vi "Get Descriptor.vi"(0 "VISA resource name":refnum<visa-resource-name>, 5 "Source (1: Channel 1)":u16(ring)=1 items=["Channel 1"=1, "Channel 2"=2, "Channel 3"=3, "Channel 4"=4], 11 "error in (no error)":errorcluster) -> (1 "First Valid Point":i32, 2 "Last Valid Point":i32, 3 "Horizontal interval":sgl, 4 "VISA resource name out":refnum<visa-resource-name>, 6 "Vertical gain":sgl, 8 "Horizontal Offset":dbl, 10 "Vertical offset":sgl, 12 "Number Of Data Points":i32, 13 "Trigger Time":T1, 14 "Command type":i16, 15 "error out":errorcluster)   [LabVIEW 2021, in "Siglent SDS 1000 2000 Series.lvlib"]
doc: "Get basic information about acquisition waveform from specified channel."
uses:
  <instrlib>/Siglent SDS 1000 2000 Series/Siglent SDS 1000 2000 Series.lvlib
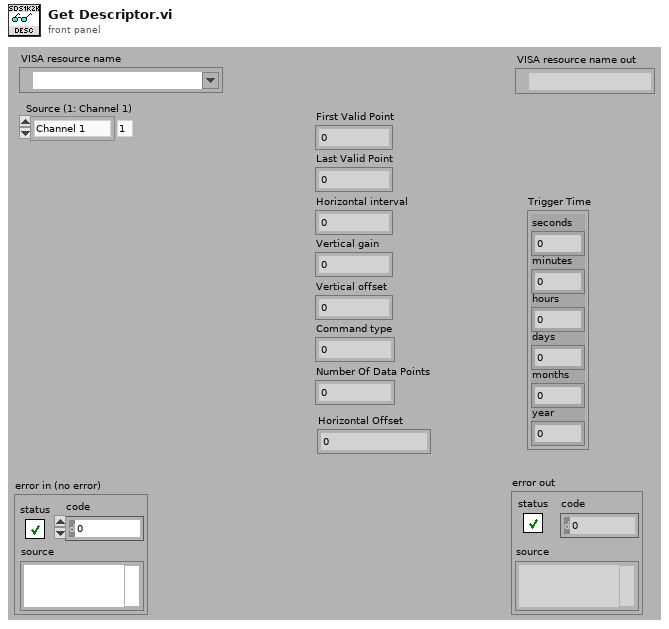
[diagram p1: front panel]
types:
  T1 = cluster{"seconds":dbl, "minutes":u8, "hours":u8, "days":u8, "months":u8, "year":u16}
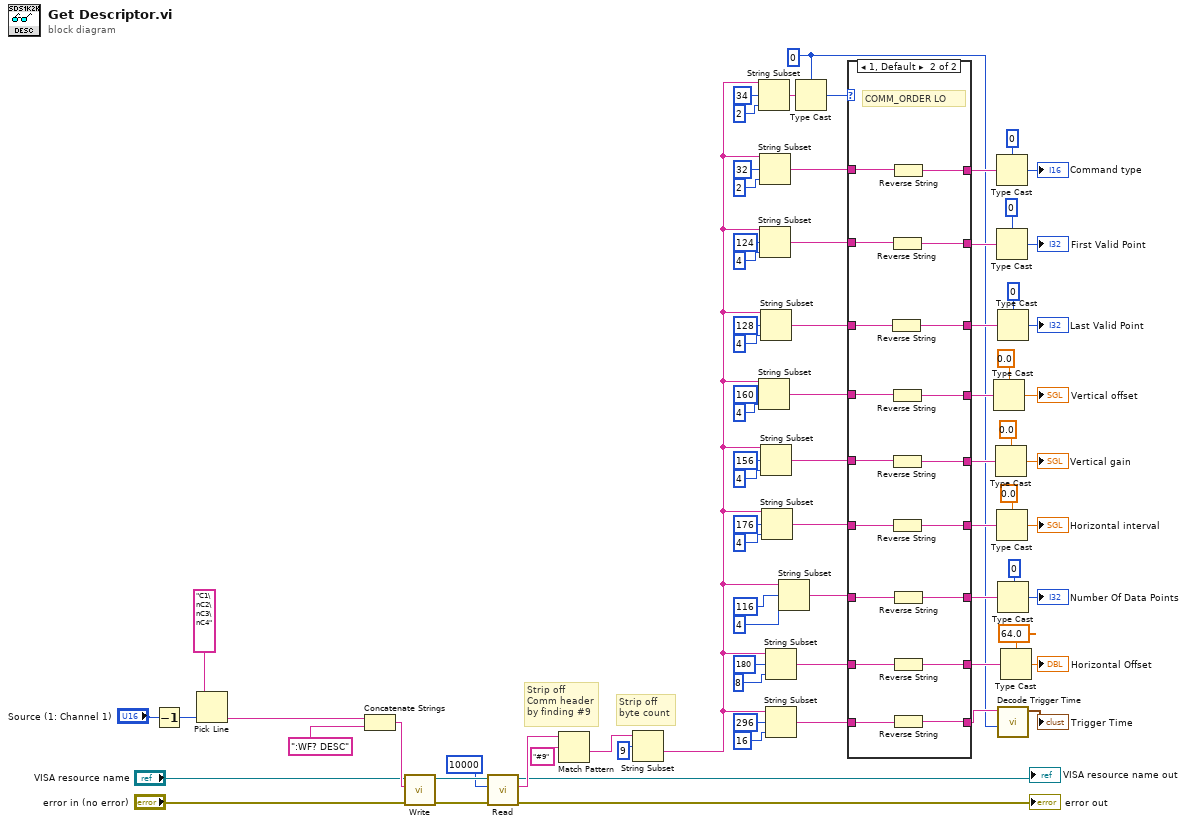
[diagram p0: block diagram]
diagram:
  w4 = i16 0
  # "Strip off byte count"
  # "Strip off\nComm header\nby finding #9"
  n1 = Decrement(x="Source (1: Channel 1)") -> (x-1=w1:u16)
  n2 = Pick Line(multi-line string="C1\nC2\nC3\nC4", line index=w1) -> (output string=w3:string)  [unwired: 1 in]
  n3 = Concatenate Strings(w3, ":WF? DESC" ("write buffer")) -> (w22:string)
  n4 = call <instrlib>:"Write.vi"("error in (no error)"="error in (no error)", "Write Buffer"=w22, "VISA resource name"="VISA resource name") -> ("error out"=w27:errorcluster, "VISA resource name out"=w20:refnum<visa-resource-name>)  [unwired: 6 in, 1 out]
  n5 = call <instrlib>:"Read.vi"("error in (no error)"=w27, "Byte Count"=u32 10000, "VISA resource name"=w20) -> ("error out"=→"error out":errorcluster, "Read Buffer"=w18:string, "VISA resource name out"=→"VISA resource name out":refnum<visa-resource-name>)  [unwired: 5 in, 1 out]
  n6 = Match Pattern(string=w18, regular expression="#9") -> (after substring=w28:string)  [unwired: 1 in, 3 out]
  n7 = String Subset(string=w28, offset (0)=9 ("length (rest)")) -> (substring=w8:string)  [unwired: 1 in]
  n8 = String Subset(string=w8, offset (0)=34, length (rest)=2 ("length (rest)")) -> (substring=w56:string)
  n9 = String Subset(string=w8, offset (0)=160, length (rest)=4 ("length (rest)")) -> (substring=w71:string)
  n10 = String Subset(string=w8, offset (0)=32, length (rest)=2 ("length (rest)")) -> (substring=w46:string)
  n11 = String Subset(string=w8, offset (0)=124, length (rest)=4 ("length (rest)")) -> (substring=w52:string)
  n12 = String Subset(string=w8, offset (0)=128, length (rest)=4 ("length (rest)")) -> (substring=w34:string)
  n13 = String Subset(string=w8, offset (0)=156, length (rest)=4 ("length (rest)")) -> (substring=w65:string)
  n14 = String Subset(string=w8, offset (0)=176, length (rest)=4 ("length (rest)")) -> (substring=w60:string)
  n15 = String Subset(string=w8, offset (0)=180, length (rest)=8 ("length")) -> (substring=w14:string)
  n16 = String Subset(string=w8, offset (0)=296, length (rest)=16 ("length (rest)")) -> (substring=w7:string)
  n17 = String Subset(string=w8, offset (0)=116, length (rest)=4 ("length (rest)")) -> (substring=w42:string)
  n18 = Type Cast(type=w4, x=w56) -> (*(type *) &x=w55:i16)
  n19 = case shown="1, Default" w55 {
    tunnel: [w85 w103] -> w72
    tunnel: w71 -> [w85 w102]
    tunnel: [w84 w101] -> w66
    tunnel: w65 -> [w84 w100]
    tunnel: [w83 w99] -> w61
    tunnel: w60 -> [w83 w98]
    tunnel: w52 -> [w82 w97]
    tunnel: [w82 w96] -> w49
    tunnel: w46 -> [w81 w91]
    tunnel: [w81 w90] -> w44
    tunnel: [w80 w94] -> w41
    tunnel: w42 -> [w80 w95]
    tunnel: w34 -> [w79 w93]
    tunnel: [w79 w92] -> w33
    tunnel: w14 -> [w78 w89]
    tunnel: [w78 w88] -> w13
    tunnel: w7 -> [w77 w87]
    tunnel: [w77 w86] -> w6
    frame 0 {
      # "COMM_ORDER HI"
    }
    frame 1, Default {
      # "COMM_ORDER LO"
      n20 = Reverse String(1:w93) -> (0:w92:string)
      n21 = Reverse String(1:w97) -> (0:w96:string)
      n22 = Reverse String(1:w102) -> (0:w103:string)
      n23 = Reverse String(1:w100) -> (0:w101:string)
      n24 = Reverse String(1:w98) -> (0:w99:string)
      n25 = Reverse String(1:w91) -> (0:w90:string)
      n26 = Reverse String(1:w95) -> (0:w94:string)
      n27 = Reverse String(1:w89) -> (0:w88:string)
      n28 = Reverse String(1:w87) -> (0:w86:string)
    }
  }
  n29 = Type Cast(type=sgl 0.0, x=w72) -> (*(type *) &x=→"Vertical offset":sgl)
  n30 = Type Cast(type=sgl 0.0, x=w66) -> (*(type *) &x=→"Vertical gain":sgl)
  n31 = Type Cast(type=i16 0, x=w44) -> (*(type *) &x=→"Command type":i16)
  n32 = Type Cast(type=0, x=w49) -> (*(type *) &x=→"First Valid Point":i32)
  n33 = Type Cast(type=sgl 0.0, x=w61) -> (*(type *) &x=→"Horizontal interval":sgl)
  n34 = Type Cast(type=0, x=w33) -> (*(type *) &x=→"Last Valid Point":i32)
  n35 = Type Cast(type=0, x=w41) -> (*(type *) &x=→"Number Of Data Points":i32)
  n36 = call <instrlib>:"Decode Trigger Time.vi"("Comm Order"=w4, "Trigger Time String"=w6) -> ("Trigger Time"=→"Trigger Time":T1)  [unwired: 9 in]
  n37 = Type Cast(type=64.0, x=w13) -> (*(type *) &x=→"Horizontal Offset":dbl)
